vi "Span2WL.vi"(8 "span":dbl, 11 "center":dbl) -> (0 "stop":dbl, 3 "start":dbl)   [LabVIEW 2017]
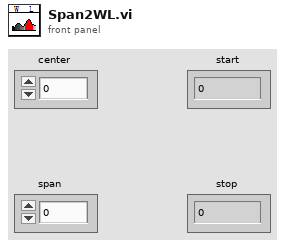
[diagram p1: front panel]
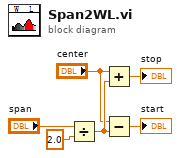
[diagram p0: block diagram]
diagram:
  n1 = Divide(x="span", y=2.0) -> (x/y=w5:dbl)
  n2 = Add(x="center", y=w5) -> (x+y=→"stop":dbl)
  n3 = Subtract(x="center", y=w5) -> (x-y=→"start":dbl)
